vi "PID_calc_AmplitudeFeedback.vi"(4 "Kd/Tau":fxp<+/-,32,6>, 5 "Ki*Tau":fxp<+/-,32,6>, 6 "Kp":fxp<+/-,32,6>, 7 "Enabled":bool=TRUE, 8 "input valid":bool=TRUE, 11 "Data in":fxp<+/-,16,14>[](array[numeric])=[0.0, 0.0, 0.0, 0.0]) -> (0 "output valid":bool, 1 "c(t) valid":bool, 2 "c(t)":fxp<+/-,32,21>, 3 "data out":fxp<+/-,16,14>[](array[numeric]))   [LabVIEW 2013]
uses:
  <vilib>/rvi/FXPMathLib/FxpDiv/subVIs/nifxpmath_Div_SimConfig.ctl
  <vilib>/rvi/FXPMathLib/FxpDiv/simVIs/DllFxpDivTemp_sub.vi
  <vilib>/rvi/FXPMathLib/FxpDiv/XNode/nifxpmath_Div.xnode
  <vilib>/rvi/FXPMathLib/FxpSub/XNode/nifxpmath_Sub.xnode
  <vilib>/rvi/FXPMathLib/FxpMul/XNode/nifxpmath_Multiplier.xnode
  <vilib>/rvi/FXPMathLib/FxpAdd/XNode/nifxpmath_Add.xnode
  <vilib>/rvi/FXPMathLib/sim/FxpSim.dll
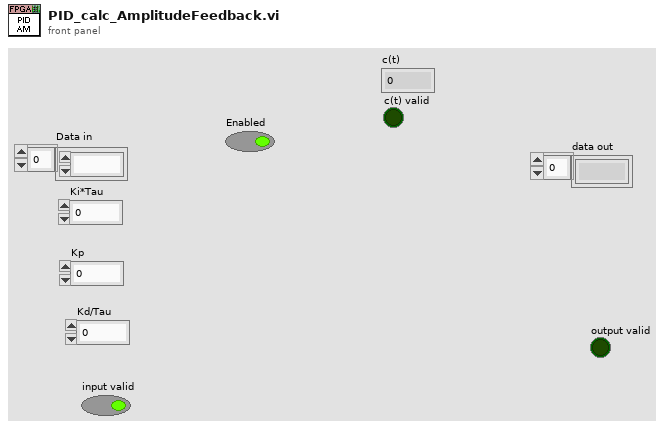
[diagram p1: front panel]
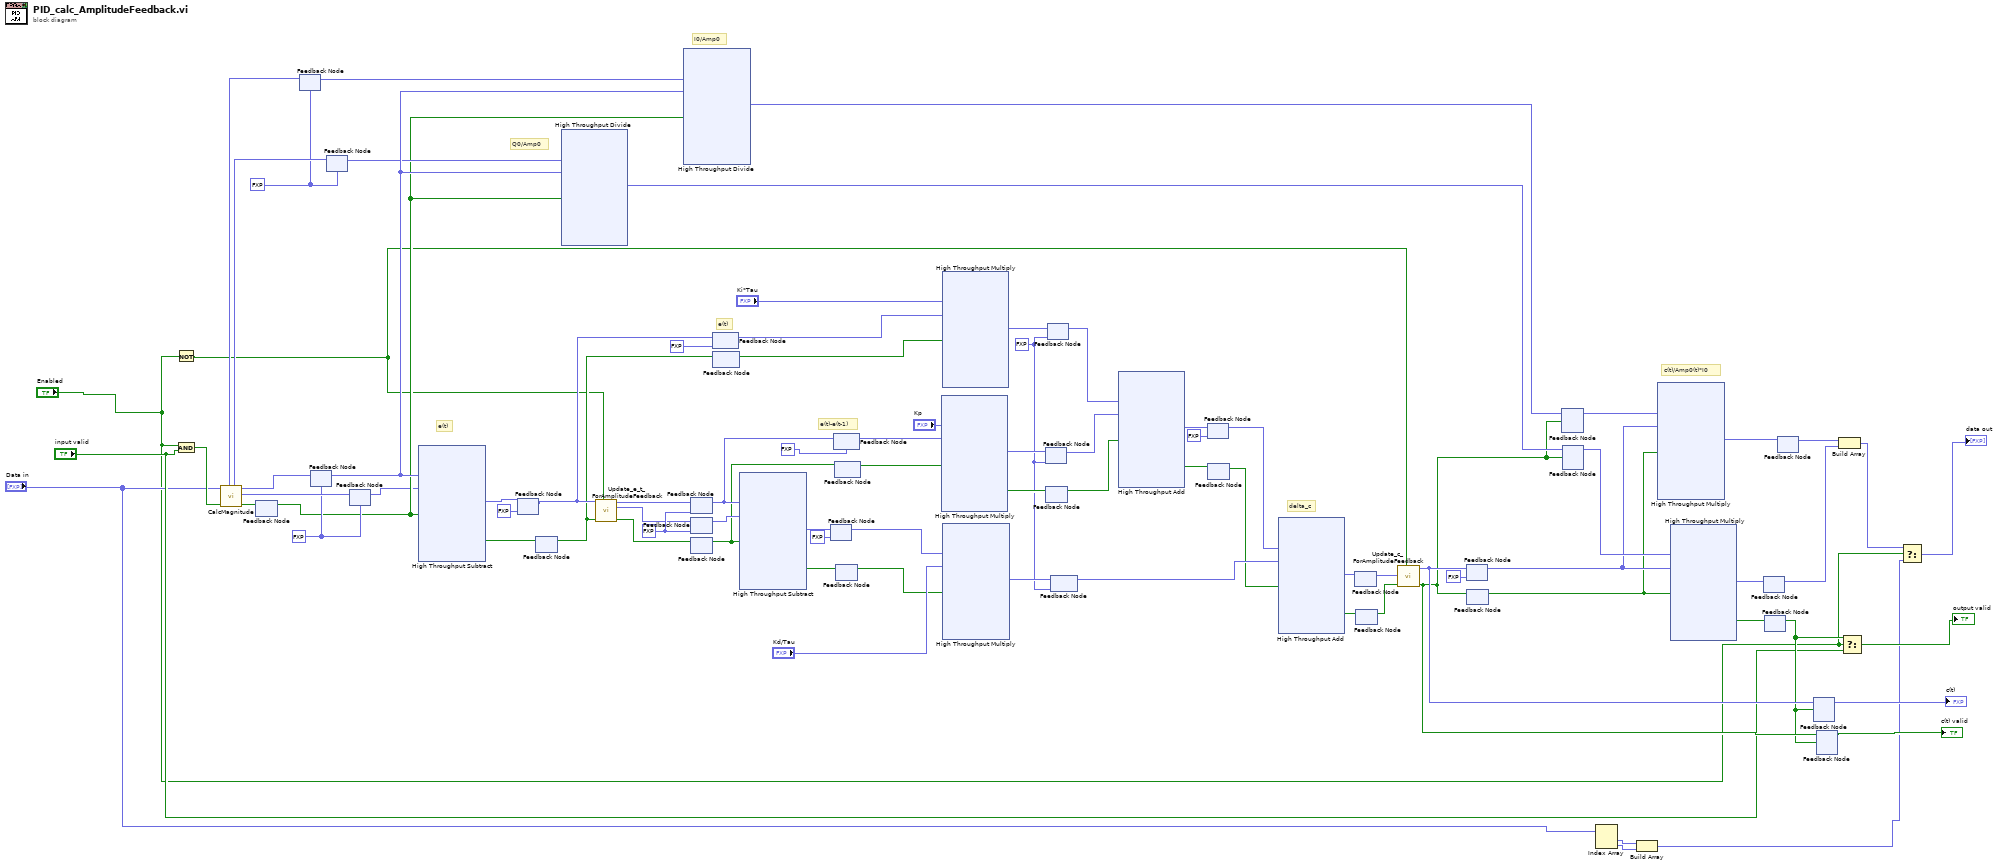
[diagram p0: block diagram]
diagram:
  w61 = fxp<+/-,32,21> 0.0 ("x*y")
  w40 = fxp<+/-,18,16> 0.0 ("e(t-1)-e(t-2)")
  w51 = fxp<+/-,16,14> 0.0 ("Q0 in")
  w57 = fxp<+,16,14> 0.0 ("Amp0")
  # "c(t)/Amp0(t)*I0"
  # "Q0/Amp0"
  # "I0/Amp0"
  # "delta_c"
  # "e(t)-e(t-1)"
  # "e(t)"
  # "e(t)"
  n1 = Not(x="Enabled") -> (.not. x?=w11:bool)
  n2 = And(x="Enabled", y="input valid") -> (x .and. y?=w24:bool)
  n3 = call "CalcMagnitude.vi"("input valid"=w24, "Data in"="Data in") -> ("output valid"=w58:bool, "Amp1"=w59:fxp<+,16,14>, "Amp0"=w60:fxp<+,16,14>, "Q0 in"=w53:fxp<+/-,16,14>, "I0 in"=w55:fxp<+/-,16,14>)  [unwired: 5 in]
  n4 = feedback #1() -> (w33:bool)  [unwired: 1 in]
  n5 = feedback-in #1(w58) -> ()
  n6 = feedback #2(w51) -> (w54:fxp<+/-,16,14>)
  n7 = feedback-in #2(w55) -> ()
  n8 = feedback #3(w57) -> (w56:fxp<+,16,14>)
  n9 = feedback-in #3(w60) -> ()
  n10 = feedback #4(w51) -> (w52:fxp<+/-,16,14>)
  n11 = feedback-in #4(w53) -> ()
  n12 = feedback #5(w57) -> (w32:fxp<+,16,14>)
  n13 = feedback-in #5(w59) -> ()
  n14 = xnode "High Throughput Subtract"("x"=w56, "y"=w32, "input valid"=w33) -> ("x-y"=w30:fxp<+/-,17,15>, "output valid"=w31:bool)  [unwired: 1 in, 1 out]
  n15 = feedback #6(fxp<+/-,17,15> 0.0 ("x-y")) -> (w15:fxp<+/-,17,15>)
  n16 = feedback-in #6(w30) -> ()
  n17 = feedback #7() -> (w14:bool)  [unwired: 1 in]
  n18 = feedback-in #7(w31) -> ()
  n19 = xnode "High Throughput Divide"("x"=w52, "y"=w56, "input valid"=w33) -> ("x/y"=w48:fxp<+/-,32,16>)  [unwired: 1 in, 2 out]
  n20 = call "Update_e_t_ForAmplitudeFeedback.vi"("Rest"=w11, "input valid"=w14, "e(t)"=w15) -> ("output valid"=w20:bool, "e(t-1)-e(t-2)"=w25:fxp<+/-,18,16>, "e(t)-e(t-1)"=w21:fxp<+/-,18,16>)  [unwired: 6 in]
  n21 = xnode "High Throughput Divide"("x"=w54, "y"=w56, "input valid"=w33) -> ("x/y"=w50:fxp<+/-,32,16>)  [unwired: 1 in, 2 out]
  n22 = feedback #8(w40) -> (w63:fxp<+/-,18,16>)
  n23 = feedback-in #8(w21) -> ()
  n24 = feedback #9(w40) -> (w82:fxp<+/-,18,16>)
  n25 = feedback-in #9(w25) -> ()
  n26 = feedback #10() -> (w62:bool)  [unwired: 1 in]
  n27 = feedback-in #10(w20) -> ()
  n28 = feedback #11(fxp<+/-,17,15> 0.0 ("x-y")) -> (w76:fxp<+/-,17,15>)
  n29 = feedback-in #11(w15) -> ()
  n30 = feedback #12() -> (w74:bool)  [unwired: 1 in]
  n31 = feedback-in #12(w14) -> ()
  n32 = xnode "High Throughput Subtract"("x"=w63, "y"=w82, "input valid"=w62) -> ("x-y"=w80:fxp<+/-,19,17>, "output valid"=w79:bool)  [unwired: 1 in, 1 out]
  n33 = feedback #13(fxp<+/-,19,17> 0.0 ("x-y")) -> (w78:fxp<+/-,19,17>)
  n34 = feedback-in #13(w80) -> ()
  n35 = feedback #14(fxp<+/-,18,16> 0.0 ("e(t-1)-e(t-2)")) -> (w23:fxp<+/-,18,16>)
  n36 = feedback-in #14(w63) -> ()
  n37 = feedback #15() -> (w22:bool)  [unwired: 1 in]
  n38 = feedback-in #15(w62) -> ()
  n39 = feedback #16() -> (w75:bool)  [unwired: 1 in]
  n40 = feedback-in #16(w79) -> ()
  n41 = xnode ("High Throughput Multiply")("x"="Kp", "y"=w23, "input valid"=w22) -> ("x*y"=w71:fxp<+/-,32,21>, "output valid"=w70:bool)  [unwired: 1 in, 1 out]
  n42 = xnode ("High Throughput Multiply")("x"="Ki*Tau", "y"=w76, "input valid"=w74) -> ("x*y"=w73:fxp<+/-,32,21>)  [unwired: 1 in, 2 out]
  n43 = xnode ("High Throughput Multiply")("x"=w78, "y"="Kd/Tau", "input valid"=w75) -> ("x*y"=w69:fxp<+/-,32,21>)  [unwired: 1 in, 2 out]
  n44 = feedback #17(w61) -> (w19:fxp<+/-,32,21>)
  n45 = feedback-in #17(w71) -> ()
  n46 = feedback #18() -> (w18:bool)  [unwired: 1 in]
  n47 = feedback-in #18(w70) -> ()
  n48 = feedback #19(w61) -> (w72:fxp<+/-,32,21>)
  n49 = feedback-in #19(w73) -> ()
  n50 = feedback #20(w61) -> (w68:fxp<+/-,32,21>)
  n51 = feedback-in #20(w69) -> ()
  n52 = xnode ("High Throughput Add")("x"=w72, "y"=w19, "input valid"=w18) -> ("x+y"=w67:fxp<+/-,32,21>, "output valid"=w66:bool)  [unwired: 1 in, 1 out]
  n53 = feedback #21(fxp<+/-,32,21> 0.0 ("x+y")) -> (w65:fxp<+/-,32,21>)
  n54 = feedback-in #21(w67) -> ()
  n55 = feedback #22() -> (w64:bool)  [unwired: 1 in]
  n56 = feedback-in #22(w66) -> ()
  n57 = xnode ("High Throughput Add")("x"=w65, "y"=w68, "input valid"=w64) -> ("x+y"=w27:fxp<+/-,32,21>, "output valid"=w26:bool)  [unwired: 1 in, 1 out]
  n58 = feedback #23() -> (w17:fxp<+/-,32,21>)  [unwired: 1 in]
  n59 = feedback-in #23(w27) -> ()
  n60 = feedback #24() -> (w16:bool)  [unwired: 1 in]
  n61 = feedback-in #24(w26) -> ()
  n62 = call "Update_c_ForAmplitudeFeedback.vi"("Reset"=w11, "input valid"=w16, "delta_c"=w17) -> ("output valid"=w12:bool, "c out"=w13:fxp<+/-,32,21>)  [unwired: 7 in]
  n63 = feedback #25(fxp<+/-,32,21> 0.0 ("c out")) -> (w29:fxp<+/-,32,21>)
  n64 = feedback-in #25(w13) -> ()
  n65 = feedback #26() -> (w28:bool)  [unwired: 1 in]
  n66 = feedback-in #26(w12) -> ()
  n67 = feedback #27() -> (w49:fxp<+/-,32,16>)  [unwired: 1 in]
  n68 = feedback-in #27(w50, w12) -> ()
  n69 = feedback #28() -> (w47:fxp<+/-,32,16>)  [unwired: 1 in]
  n70 = feedback-in #28(w48, w12) -> ()
  n71 = Index Array(array="Data in") -> (element #1=w7:fxp<+/-,16,14>, element #2=w1:fxp<+/-,16,14>)  [unwired: 2 in]
  n72 = Build Array(w7, w1) -> (w3:fxp<+/-,16,14>[])
  n73 = xnode ("High Throughput Multiply")("x"=w49, "y"=w29, "input valid"=w28) -> ("x*y"=w46:fxp<+/-,16,14>)  [unwired: 1 in, 2 out]
  n74 = xnode ("High Throughput Multiply")("x"=w47, "y"=w29, "input valid"=w28) -> ("x*y"=w45:fxp<+/-,16,14>, "output valid"=w44:bool)  [unwired: 1 in, 1 out]
  n75 = feedback #29() -> (w42:fxp<+/-,16,14>)  [unwired: 1 in]
  n76 = feedback-in #29(w45) -> ()
  n77 = feedback #30() -> (w10:bool)  [unwired: 1 in]
  n78 = feedback-in #30(w44) -> ()
  n79 = feedback #31() -> (w43:fxp<+/-,16,14>)  [unwired: 1 in]
  n80 = feedback-in #31(w46) -> ()
  n81 = feedback #32() -> (→"c(t)":fxp<+/-,32,21>)  [unwired: 1 in]
  n82 = feedback-in #32(w13, w10) -> ()
  n83 = feedback #33() -> (→"c(t) valid":bool)  [unwired: 1 in]
  n84 = feedback-in #33(w12, w10) -> ()
  n85 = Build Array(w43, w42) -> (w5:fxp<+/-,16,14>[])
  n86 = Select(t=w10, s="Enabled", f="input valid") -> (s? t:f=→"output valid":bool)
  n87 = Select(t=w5, s="Enabled", f=w3) -> (s? t:f=→"data out":fxp<+/-,16,14>[])
